vi "readHSdata.vi"(8 "error in (no error)":errorcluster, 10 "HS Loop AI":fxp<+/-,25,5>[](array[numeric])=[0.0, 0.0, 0.0, 0.0]) -> (0 "error out":errorcluster, 3 "PositionMeas out":refnum<class "PositionMeas.lvclass">)   [LabVIEW 2020, in "PositionMeas.lvclass"]
doc: "Update data from the High-Speed AI loop and store it in the PositionMeas data storage"
uses:
  PositionMeas.lvclass
  PositionMeas.lvclass/PositionMeas.ctl
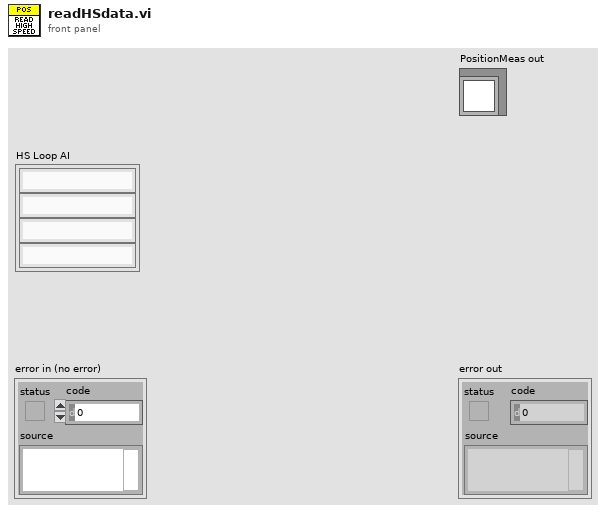
[diagram p1: front panel]
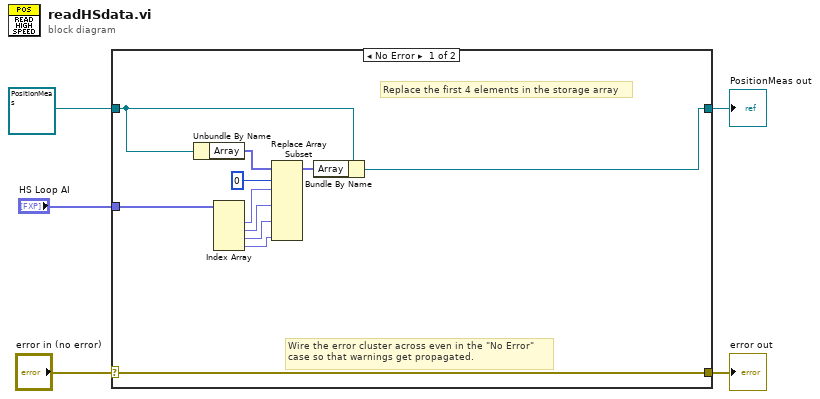
[diagram p0: block diagram]
diagram:
  n1 = case shown="No Error" "error in (no error)" {
    selector: "error in (no error)" -> [w16 w18]
    tunnel: [w16 w18] -> w4
    tunnel: [w6 w17] -> w3
    tunnel: refnum<class "PositionMeas.lvclass"> refnum ("PositionMeas.lvclass") -> [w14 w17]
    tunnel: "HS Loop AI" -> [w12 _]
    frame No Error {
      # "Replace the first 4 elements in the storage array"
      # "Wire the error cluster across even in the \"No Error\"\ncase so that warnings get propagated."
      n2 = Unbundle By Name(w14) -> ("Array"=w15:fxp<+/-,25,5>[])
      n3 = Index Array(array=w12) -> (element #1=w11:fxp<+/-,25,5>, element #2=w10:fxp<+/-,25,5>, element #3=w9:fxp<+/-,25,5>, element #4=w8:fxp<+/-,25,5>)  [unwired: 4 in]
      n4 = Replace Array Subset(array=w15, new element #1=w11, index #1=0 ("index"), new element #2=w10, new element #3=w9, new element #4=w8) -> (w7:fxp<+/-,25,5>[])  [unwired: 3 in]
      n5 = Bundle By Name(cluster=w14, "Array"=w7) -> (w6:refnum<class "PositionMeas.lvclass">)
    }
    frame Error {
    }
  }
  "error out" <- w4
  "PositionMeas out" <- w3
